vi "Sec to Time Str.vi"(0 "Time s":dbl) -> (4 "String":string)   [LabVIEW 2019]
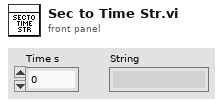
[diagram p1: front panel]
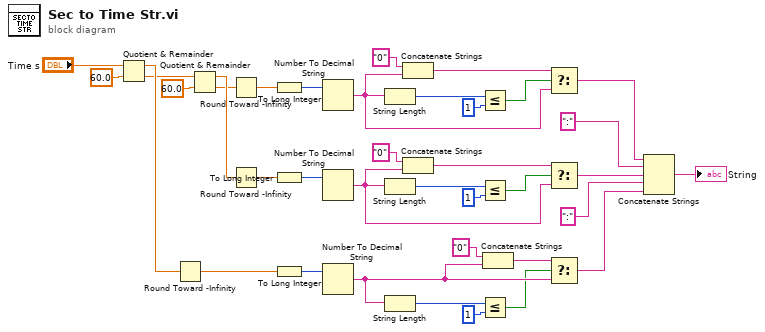
[diagram p0: block diagram]
diagram:
  n1 = Quotient & Remainder(x="Time s", y=60.0) -> (x-y*floor(x/y)=w24:dbl, floor(x/y)=w20:dbl)
  n2 = Round Toward -Infinity(1:w24) -> (0:w25:dbl)
  n3 = Quotient & Remainder(x=w20, y=60.0) -> (x-y*floor(x/y)=w19:dbl, floor(x/y)=w16:dbl)
  n4 = Round Toward -Infinity(1:w16) -> (0:w17:dbl)
  n5 = Round Toward -Infinity(1:w19) -> (0:w34:dbl)
  n6 = To Long Integer(number=w17) -> (32bit integer=w18:i32)
  n7 = To Long Integer(number=w34) -> (32bit integer=w33:i32)
  n8 = To Long Integer(number=w25) -> (32bit integer=w26:i32)
  n9 = Number To Decimal String(number=w18) -> (decimal integer string=w2:string)  [unwired: 1 in]
  n10 = Number To Decimal String(number=w33) -> (decimal integer string=w9:string)  [unwired: 1 in]
  n11 = Number To Decimal String(number=w26) -> (decimal integer string=w32:string)  [unwired: 1 in]
  n12 = String Length(string=w2) -> (length=w3:i32)
  n13 = String Length(string=w9) -> (length=w14:i32)
  n14 = String Length(string=w32) -> (length=w27:i32)
  n15 = Concatenate Strings("0" ("string"), w2) -> (w7:string)
  n16 = Concatenate Strings("0" ("string"), w9) -> (w10:string)
  n17 = Less Or Equal?(x=w3, y=1) -> (x <= y?=w5:bool)
  n18 = Less Or Equal?(x=w14, y=1) -> (x <= y?=w12:bool)
  n19 = Less Or Equal?(x=w27, y=1) -> (x <= y?=w29:bool)
  n20 = Concatenate Strings("0" ("string"), w32) -> (w31:string)
  n21 = Select(t=w7, s=w5, f=w2) -> (s? t:f=w1:string)
  n22 = Select(t=w10, s=w12, f=w9) -> (s? t:f=w8:string)
  n23 = Select(t=w31, s=w29, f=w32) -> (s? t:f=w36:string)
  n24 = Concatenate Strings(w1, ":" ("string"), w8, ":" ("string"), w36) -> (→"String":string)
